vi "Score.vi"(7 "Mov_Spd":i32=5, 8 "error in":errorcluster, 10 "Obs D_in":refnum<vi>[](array[refnum]), 11 "Ball in":refnum<vi>) -> (0 "error out":errorcluster, 2 "Msg":string, 3 "Add":i32)   [LabVIEW 2012]
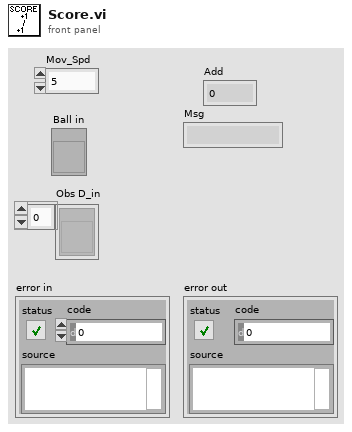
[diagram p1: front panel]
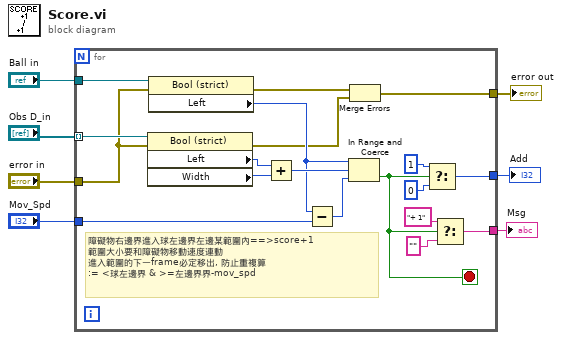
[diagram p0: block diagram]
diagram:
  n1 = for {
    tunnel: "Mov_Spd" -> [w26]
    tunnel: [w22] -> w6
    tunnel: "Ball in" -> [w15]
    tunnel: "Obs D_in" -> [w14] mode=indexing
    tunnel: [w13] -> w4
    tunnel: "error in" -> [w12]
    tunnel: [w10] -> w1
    stop <- w11 stop-if-true
    # "障礙物右邊界進入球左邊界左邊某範圍內==>score+1\n範圍大小要和障礙物移動速度連動\n進入範圍的下一frame必定移出, 防止重複算\n:= <球左邊界 & >=左邊界界-mov_spd"
    n2 = property on="Property Node" class="Bool (strict)"(reference=w14, error in=w12) -> (error out=w20:errorcluster, "Left"=w19:i32, "Width"=w18:u32)  [unwired: 1 out]
    n3 = property on="Property Node" class="Bool (strict)"(reference=w15, error in=w12) -> (error out=w21:errorcluster, "Left"=w23:i32)  [unwired: 1 out]
    n4 = Add(x=w19, y=w18) -> (x+y=w25:u32)
    n5 = Subtract(x=w23, y=w26) -> (x-y=w24:i32)
    n6 = In Range and Coerce(upper limit=w23, x=w25, lower limit=w24) -> (In Range?=w11:bool)  [unwired: 1 out]
    n7 = Merge Errors(w21, w20) -> (w13:errorcluster)
    n8 = Select(t=1, s=w11, f=0 ("t")) -> (s? t:f=w22:i32)
    n9 = Select(t="+ 1", s=w11, f="") -> (s? t:f=w10:string)
  }
  "Add" <- w6
  "error out" <- w4
  "Msg" <- w1
